vi "Insert Results into Excel lookup column.vi"(0 "report in":refnum<class "NI_report.lvclass">, 1 "strings":string[](array[string]), 2 "Pass/Fail":bool[](array[boolean]), 5 "columns":i32[](array[numeric]), 7 "row":i32, 11 "error in":errorcluster) -> (4 "report out":refnum<class "NI_report.lvclass">, 6 "column out":i32, 15 "error out":errorcluster)   [LabVIEW 2015]
uses:
  <vilib>/Utility/NIReport.llb/NI_report.lvclass
  <vilib>/Utility/NIReport.llb/Append Report Text (str wrap).vi
  <vilib>/Utility/NIReport.llb/Excel/NI_Excel.lvclass
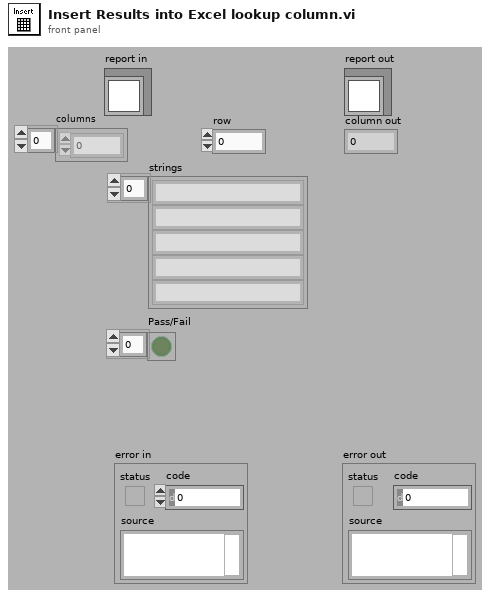
[diagram p1: front panel]
types:
  T1 = cluster{"position (excel)":cluster{"row":i32, "column":i32}, "name (excel)":string, "bookmark (word)":string}
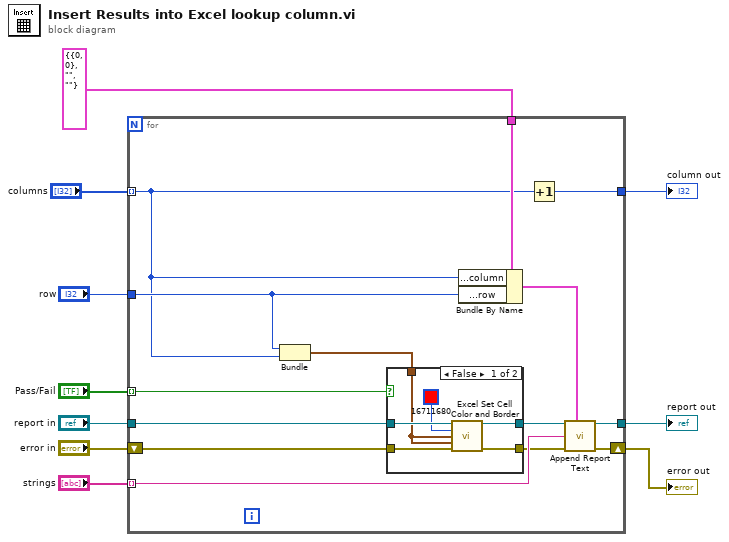
[diagram p0: block diagram]
diagram:
  n1 = for {
    tunnel: "strings" -> [w24] mode=indexing
    tunnel: "report in" -> [w12]
    tunnel: [w23] -> w3
    tunnel: T1 {"position (excel)"={"row"=0, "column"=0}, "name (excel)"="", "bookmark (word)"=""} ("MS Office parameters") -> [w21]
    tunnel: "row" -> [w16]
    shift-right: [w22] -> w2
    shift-left: "error in" -> [w13]
    tunnel: "Pass/Fail" -> [w14] mode=indexing
    tunnel: [w19] -> w5
    tunnel: "columns" -> [w11] mode=indexing
    n2 = Bundle("row"=w16, "column"=w11) -> (w15:cluster{"row":i32, "column":i32})  [unwired: 1 in]
    n3 = case shown="False" w14 {
      tunnel: [w30 w32] -> w18
      tunnel: [w29 w31] -> w17
      tunnel: w12 -> [w28 w32]
      tunnel: w13 -> [w27 w31]
      tunnel: w15 -> [w26 _]
      frame False {
        n4 = call <vilib>:"Excel Set Cell Color and Border.vi"("report in"=w28, "background color (w)"=u32 16711680, "start (-1, -1)"=w26, "end (-1, -1)"=w26, "error in (no error)"=w27) -> ("report out"=w30:refnum<class "NI_report.lvclass">, "error out"=w29:errorcluster)  [unwired: 9 in]
      }
      frame True {
      }
    }
    n5 = Bundle By Name(cluster=w21, "position (excel).column"=w11, "position (excel).row"=w16) -> (w20:T1)
    n6 = Increment(x=w11) -> (x+1=w19:i32)
    n7 = call-poly <vilib>:"Append Report Text.vi"("report in"=w18, "MS Office parameters"=w20, "text"=w24, "error in (no error)"=w17) -> ("report out"=w23:refnum<class "NI_report.lvclass">, "error out"=w22:errorcluster)  [unwired: 8 in, 2 out]
  }
  "error out" <- w2
  "column out" <- w5
  "report out" <- w3
